vi "LIN EX Master Sync.vi"(6 "MsgLen":u32, 7 "pOutMsg":T1, 9 "pInMsg":T1, 10 "LINIndex":u8, 11 "DevHandle":i32) -> (1 "pInMsg out":T1, 3 "function return":i32, 5 "pOutMsg out":T1)   [LabVIEW 2010, in "usb2lin_ex.lvlib"]
doc: "int WINAPI LIN_EX_MasterSync(int DevHandle,unsigned char LINIndex,LIN_EX_MSG *pInMsg,LIN_EX_MSG *pOutMsg,unsigned int MsgLen);"
uses:
  usb2lin_ex.lvlib
  USB2XXX.dll
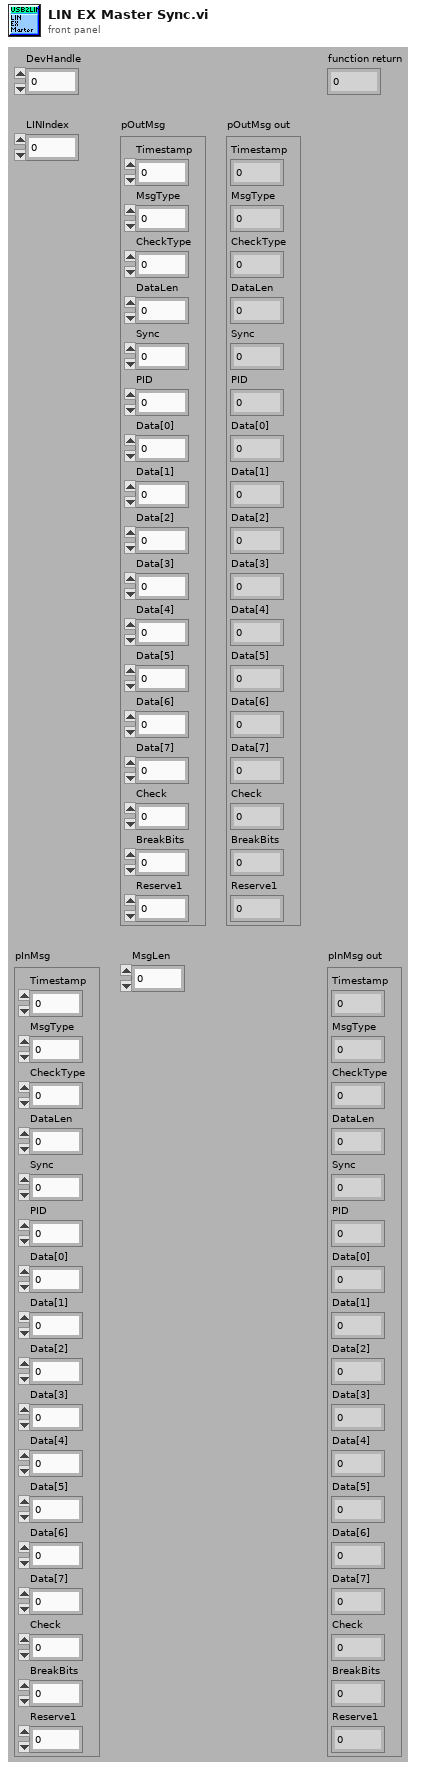
[diagram p1: front panel]
types:
  T1 = cluster{"Timestamp":u32, "MsgType":u8, "CheckType":u8, "DataLen":u8, "Sync":u8, "PID":u8, "Data[0]":u8, "Data[1]":u8, "Data[2]":u8, "Data[3]":u8, "Data[4]":u8, "Data[5]":u8, "Data[6]":u8, "Data[7]":u8, "Check":u8, "BreakBits":u8, "Reserve1":u8}
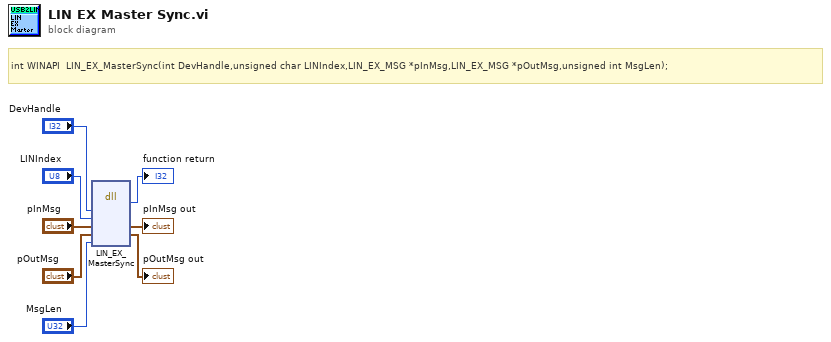
[diagram p0: block diagram]
diagram:
  # "int WINAPI  LIN_EX_MasterSync(int DevHandle,unsigned char LINIndex,LIN_EX_MSG *pInMsg,LIN_EX_MSG *pOutMsg,unsigned int MsgLen);"
  n1 = dll-call lib="E:/OtherWork/STM32/USB2XXX_Example/sdk/api/Labview/USB2XXX.*" fn="LIN_EX_MasterSync"("DevHandle"="DevHandle", "LINIndex"="LINIndex", "pInMsg"="pInMsg", "pOutMsg"="pOutMsg", "MsgLen"="MsgLen") -> (→"function return":i32, "pInMsg"=→"pInMsg out":T1, "pOutMsg"=→"pOutMsg out":T1)  [unwired: 6 in, 2 out]
